vi "军蚁-工具栏按钮操作.vi"(8 "error in (no error)":errorcluster caption="错误输入（无错误）", 9 "布尔":bool=TRUE, 10 "禁用":T1(ring), 11 "引用数组":refnum<vi>[](array[refnum])) -> (0 "error out":errorcluster caption="错误输出")   [LabVIEW 2017]
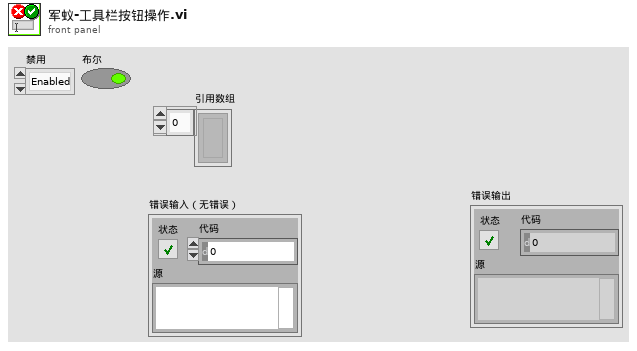
[diagram p1: front panel]
types:
  T1 = enum8{"Enabled", "Disabled", "Disabled and Grayed Out"}
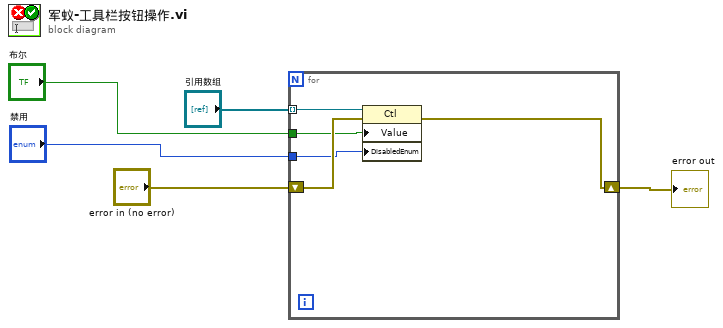
[diagram p0: block diagram]
diagram:
  n1 = for {
    tunnel: "引用数组" -> [w10] mode=indexing
    shift-right: [w8] -> w3
    shift-left: "error in (no error)" -> [w9]
    tunnel: "禁用" -> [w7]
    tunnel: "布尔" -> [w6]
    n2 = property class="Ctl"(reference=w10, error in=w9, "Value"=w6, "DisabledEnum"=w7) -> (error out=w8:errorcluster)  [unwired: 1 out]
  }
  "error out" <- w3
